vi "options.vi"(9 "server information":T1, 10 "application request in":T4, 11 "test responder in":refnum<class "test responder.lvclass">) -> (2 "application response out":T2, 3 "test responder out":refnum<class "test responder.lvclass">)   [LabVIEW 2016, in "test responder.lvclass"]
uses:
  test responder.lvclass
  HTTP server/http request.ctl
  HTTP server/http method.ctl
  HTTP headers/http header data.ctl
  HTTP server/http response.ctl
  HTTP server/http server info.ctl
  HTTP responder/https responder.lvclass
  HTTP server/Basic HTTPS server.lvclass
  HTTP headers/http headers.lvlib
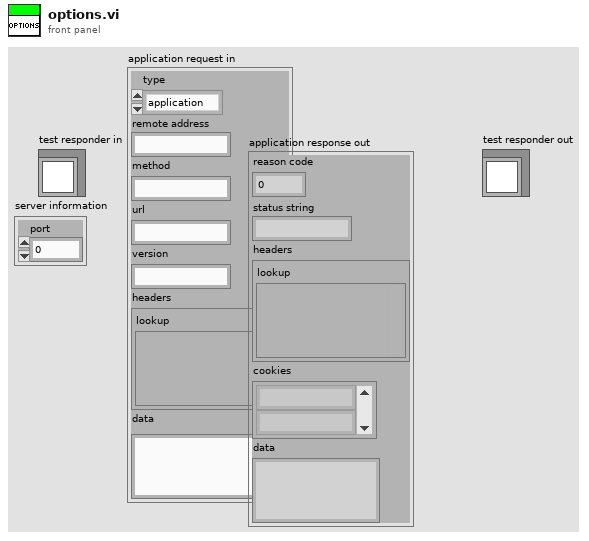
[diagram p1: front panel]
types:
  T1 = typedef "Basic HTTPS server.lvclass/http server info.ctl" = cluster{"port":u16}
  T2 = typedef "Basic HTTPS server.lvclass/http response.ctl" = cluster{"reason code":u16, "status string":string, "headers":T3, "cookies":string[], "data":string}
  T3 = typedef "http headers.lvlib/http header data.ctl" = cluster{"lookup":variant}
  T4 = typedef "Basic HTTPS server.lvclass/http request.ctl" = cluster{"type":T5, "remote address":string, "method":string, "url":string, "version":string, "headers":T3, "data":string}
  T5 = typedef "Basic HTTPS server.lvclass/http method.ctl" = enum16{"application", "error", "upgrade"}
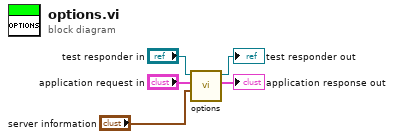
[diagram p0: block diagram]
diagram:
  n1 = call-parent "options.vi"("server information"="server information", "application request in"="application request in", "http responder in"="test responder in") -> ("application response out"=→"application response out":T2, "http responder out"=→"test responder out":refnum<class "test responder.lvclass">)  [unwired: 7 in]
